vi "GT_Close.vi"(1 "rtn_In":cluster{"rtn":i16, "Func":string}) -> (0 "rtn_Out":cluster{"rtn":i16, "Func":string})   [LabVIEW 2014]
uses:
  VC6/gts.dll
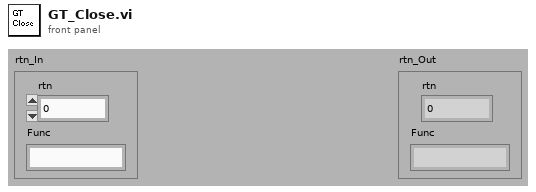
[diagram p1: front panel]
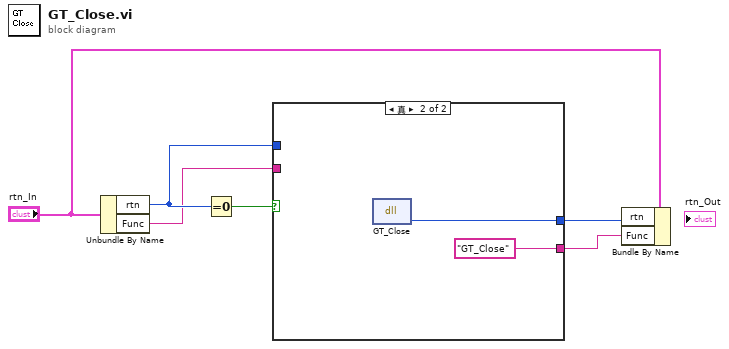
[diagram p0: block diagram]
diagram:
  n1 = Unbundle By Name("rtn_In") -> ("rtn"=w5:i16, "Func"=w4:string)
  n2 = Equal To 0?(x=w5) -> (x = 0?=w6:bool)
  n3 = case shown="真" w6 {
    tunnel: w5 -> [w8 _]
    tunnel: w4 -> [w7 _]
    tunnel: [w8 w10] -> w2
    tunnel: [w7 "GT_Close" ("Func")] -> w1
    frame False {
    }
    frame True {
      n4 = dll-call lib="PTH2Iabs E+Win7系统AC-800标准版源程序-20170822gts85VC6gts.dll" fn="GT_Close"() -> ("rtn"=w10:i16)  [unwired: 3 in, 2 out]
    }
  }
  n5 = Bundle By Name(cluster="rtn_In", "rtn"=w2, "Func"=w1) -> ()  [unwired: 1 out]
